vi "Ball_num_var.vi"() -> ()   [LabVIEW 2019]
panel:
  in  "Ball num":dbl
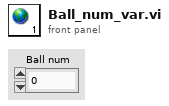
[diagram p1: front panel]
diagram:
